vi "get subresults.vi"(8 "error in":errorcluster, 11 "result in":refnum<class "result.lvclass">) -> (0 "error out":errorcluster, 2 "subresults":refnum<class "result.lvclass">[](array[class]), 3 "result out":refnum<class "result.lvclass">)   [LabVIEW 2013, in "result.lvclass"]
uses:
  result.lvclass
  result.lvclass/result.ctl
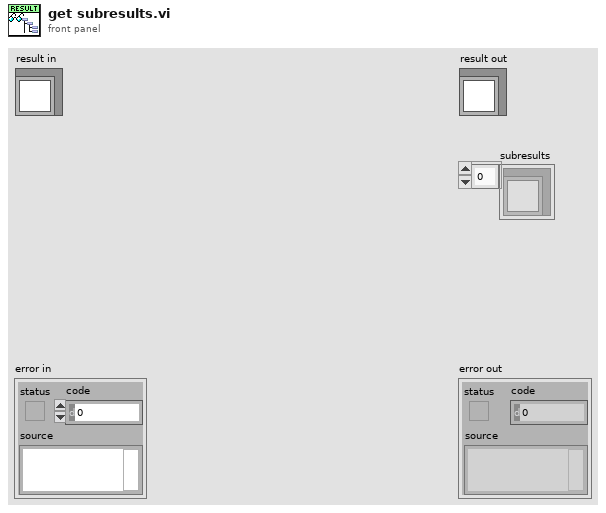
[diagram p1: front panel]
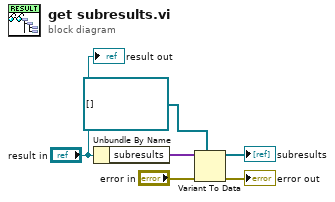
[diagram p0: block diagram]
diagram:
  n1 = Unbundle By Name("result in") -> ("subresults"=w2:variant[])
  n2 = Variant To Data(error in="error in", type=refnum<class "result.lvclass">[] [], Variant=w2) -> (data=→"subresults":refnum<class "result.lvclass">[], error out=→"error out":errorcluster)
  "result out" <- "result in"
